vi "evenoddsubvi.vi"(1 "x":dbl) -> (0 "s? t:f":string)   [LabVIEW 2019]
doc: "THIS SUB VI WILL GIVE INFORMATION ABOUT NUMBER WETHER IT IS EVEN OR ODD."
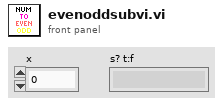
[diagram p1: front panel]
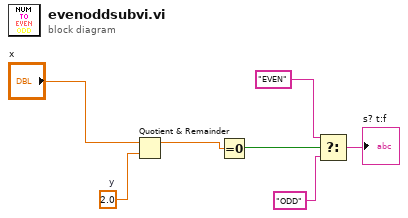
[diagram p0: block diagram]
diagram:
  w2 = 2.0  # y
  n1 = Quotient & Remainder(x="x", y=w2) -> (x-y*floor(x/y)=w3:dbl)  [unwired: 1 out]
  n2 = Equal To 0?(x=w3) -> (x = 0?=w4:bool)
  n3 = Select(t="EVEN", s=w4, f="ODD") -> (s? t:f=→"s? t:f":string)
